vi "test Add-Find-Remove.vi"(8 "error in":errorcluster, 11 "TestCase in":refnum<class "Scripting.lvclass">) -> (0 "error out":errorcluster, 3 "TestCase out":refnum<class "Scripting.lvclass">)   [LabVIEW 2020, in "Scripting.lvclass"]
uses:
  Scripting.lvclass
  <vilib>/NI VeriStand/Custom Device API/Custom Device Item Ref.ctl
  Shared/Direction.ctl
  Shared/SDI.ctl
  Scripting.lvclass/Scripting.ctl
  Shared/Transfer Type.ctl
  <vilib>/addons/_JKI Toolkits/VI Tester/TestCase.llb/TestCase.lvclass
  Scripting/AIM/AIM ARINC 429 Scripting.lvlib
  <vilib>/NI VeriStand/Custom Device API/Custom Device API.lvlib
  C:/Program Files (x86)/National Instruments/LabVIEW 2020/vi.lib/addons/_JKI Toolkits/VI Tester/TestCase.llb/TestCase.lvclass
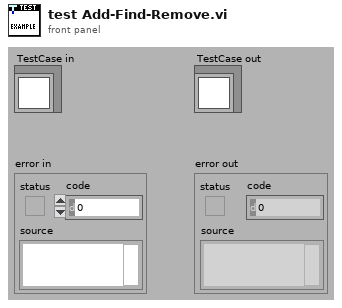
[diagram p1: front panel]
types:
  T1 = typedef "Direction.ctl" = enum16{"Rx", "Tx"}
  T2 = typedef "Custom Device API.lvlib/Custom Device Item Ref.ctl" = u64
  T3 = typedef "Transfer Type.ctl" = enum16{"Scheduled", "Acyclic", "Block", "Strobe"}
  T4 = typedef "SDI.ctl" = i32
  T5 = typedef "Custom Device API.lvlib/Custom Device Item Info.ctl" = cluster{"Name":string, "Is Channel":bool, "GUID":string, "Is Waveform":bool}
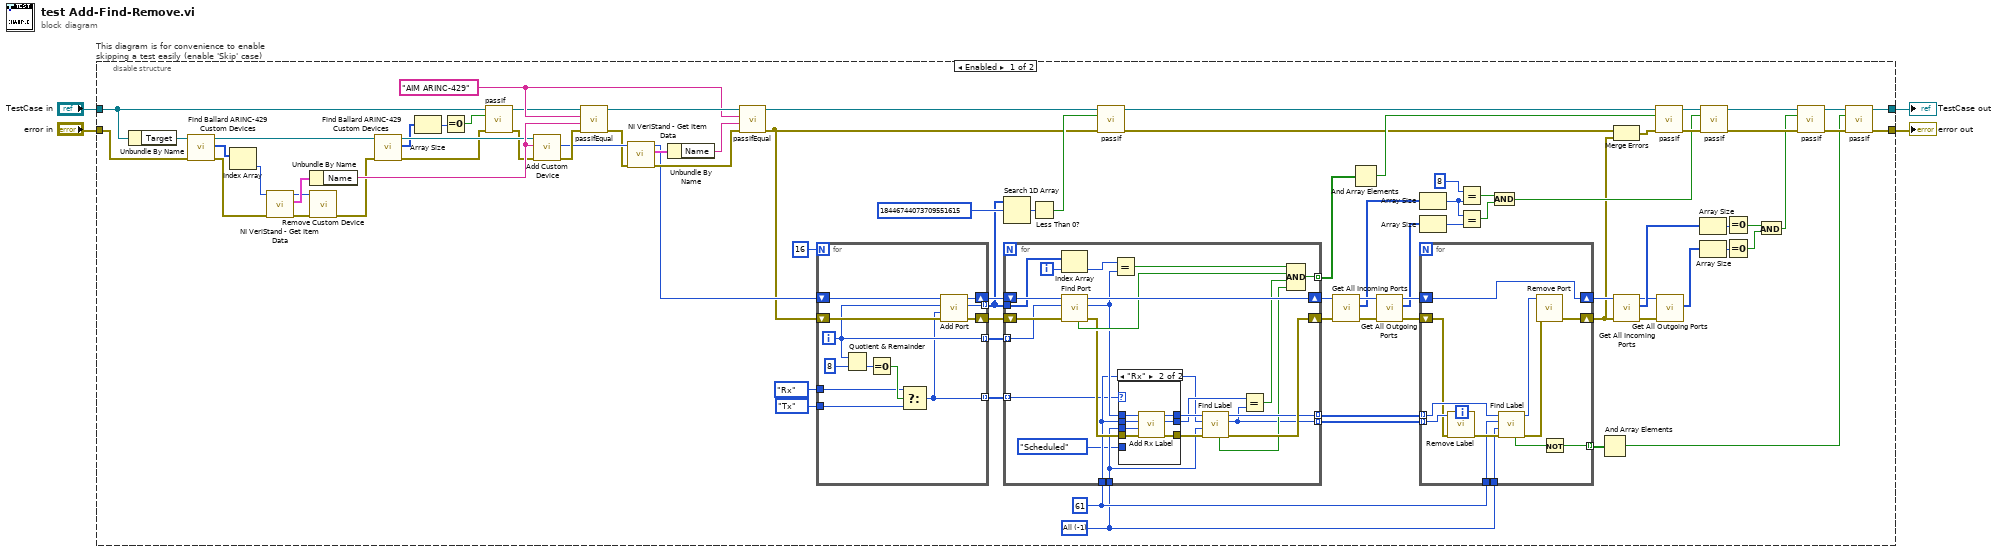
[diagram p0: block diagram]
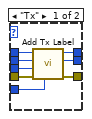
[diagram p2: hidden frame]
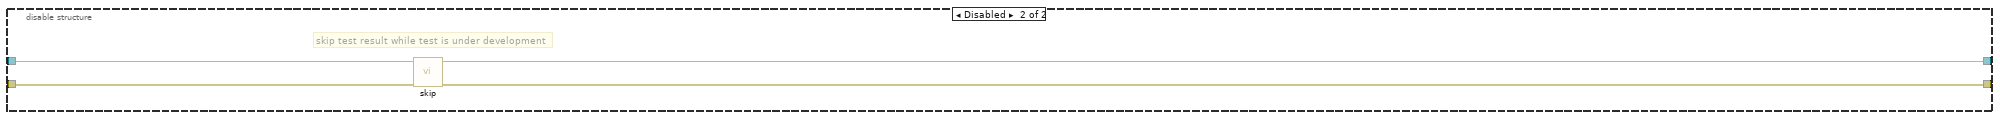
[diagram p3: hidden frame]
diagram:
  n1 = disable-structure "This diagram is for convenience to enable skipping a test easily (enable 'Skip' case)" shown="Enabled" {
    disable-tunnel: "TestCase in" -> [w69 w156]
    disable-tunnel: [w7 w154] -> w1
    disable-tunnel: [w8 w155] -> w3
    disable-tunnel: "error in" -> [w87 w153]
    frame Enabled {
      w13 = u32 61 ("label value")
      w12 = T4 -1 items=["All"=-1, "0 (b00)"=0, "1 (b01)"=1, "2 (b10)"=2, "3 (b11)"=3] ("SDI value")
      w75 = "AIM ARINC-429" ("string")
      n2 = Unbundle By Name(w69) -> ("Target"=w89:refnum<k24>)
      n3 = call "Find Ballard ARINC-429 Custom Devices.vi"("error in"=w87, "target in"=w89) -> ("error out"=w84:errorcluster, "AIM ARINC 429 custom devices"=w86:u64[], "target out"=w72:refnum<k24>)  [unwired: 7 in]
      n4 = Index Array(array=w86) -> (element=w85:u64)  [unwired: 1 in]
      n5 = call <vilib>:"NI VeriStand - Get Item Data.vi"("error in (no error)"=w84, "Item Ref in"=w85) -> ("error out"=w73:errorcluster, "Item Info"=w83:T5, "Item Ref out"=w74:T2)  [unwired: 6 in, 1 out]
      n6 = Unbundle By Name(w83) -> ("Name"=w77:string)
      n7 = call "Remove Custom Device.vi"("error in"=w73, "Ballard ARINC 429 custom device"=w74) -> ("error out"=w70:errorcluster)  [unwired: 9 in]
      n8 = call "Find Ballard ARINC-429 Custom Devices.vi"("error in"=w70, "target in"=w72) -> ("error out"=w68:errorcluster, "AIM ARINC 429 custom devices"=w65:u64[], "target out"=w71:refnum<k24>)  [unwired: 7 in]
      n9 = Array Size(array=w65) -> (size(s)=w64:i32)
      n10 = Equal To 0?(x=w64) -> (x = 0?=w63:bool)
      n11 = call-dynamic "passIf.vi"("error in (no error)"=w68, "pass"=w63, "TestCase in"=w69) -> ("error out"=w66:errorcluster, "TestCase out"=w67:refnum<class "Scripting.lvclass">)  [unwired: 7 in]
      n12 = call "Add Custom Device.vi"("error in"=w66, "name"=w77, "target in"=w71) -> ("error out"=w82:errorcluster, "Ballard ARINC 429 custom device"=w81:T2)  [unwired: 6 in, 1 out]
      n13 = call-dynamic "passIfEqual.vi"("error in (no error)"=w82, "y"=w77, "x"=w75, "TestCase in"=w67) -> ("error out"=w80:errorcluster, "TestCase out"=w88:refnum<class "Scripting.lvclass">)  [unwired: 6 in]
      n14 = call <vilib>:"NI VeriStand - Get Item Data.vi"("error in (no error)"=w80, "Item Ref in"=w81) -> ("error out"=w78:errorcluster, "Item Info"=w79:T5, "Item Ref out"=w62:T2)  [unwired: 6 in, 1 out]
      n15 = Unbundle By Name(w79) -> ("Name"=w76:string)
      n16 = call-dynamic "passIfEqual.vi"("error in (no error)"=w78, "y"=w76, "x"=w75, "TestCase in"=w88) -> ("error out"=w18:errorcluster, "TestCase out"=w21:refnum<class "Scripting.lvclass">)  [unwired: 6 in]
      n17 = for {
        N: 16 -> [_]
        shift-right: [w148] -> w61
        shift-left: w62 -> [w152]
        tunnel: [w147] -> w55 mode=indexing
        shift-right: [w145] -> w60
        shift-left: w18 -> [w146]
        tunnel: [w144] -> w59 mode=indexing
        tunnel: Direction."Rx" ("direction") -> [w143]
        tunnel: Direction."Tx" ("direction") -> [w142]
        tunnel: [w141] -> w5 mode=indexing
        i -> [w144]
        n18 = Quotient & Remainder(x=w144, y=8) -> (floor(x/y)=w150:i32)  [unwired: 1 out]
        n19 = Equal To 0?(x=w150) -> (x = 0?=w149:bool)
        n20 = Select(t=w143, s=w149, f=w142) -> (s? t:f=w141:T1)
        n21 = call "Add Port.vi"("error in"=w146, "direction"=w141, "port number"=w144, "Ballard ARINC 429 custom device in"=w152) -> ("error out"=w145:errorcluster, "port"=w147:T2, "Ballard ARINC 429 custom device out"=w148:T2)  [unwired: 5 in]
      }
      n22 = Search 1D Array(1D array=w55, element=T2 18446744073709551615 ("custom device ref out")) -> (index of element=w22:i32)  [unwired: 1 in]
      n23 = for {
        shift-right: [w124] -> w52
        shift-left: w61 -> [w125]
        tunnel: w59 -> [w122] mode=indexing
        tunnel: w55 -> [w119]
        shift-right: [w111] -> w51
        shift-left: w60 -> [w123]
        tunnel: [w110] -> w57 mode=indexing
        tunnel: [w116] -> w41 mode=indexing
        tunnel: [w106] -> w14 mode=indexing
        tunnel: w12 -> [w105]
        tunnel: w13 -> [w104]
        tunnel: w5 -> [w102] mode=indexing
        i -> [w121]
        n24 = Index Array(array=w119, index=w121) -> (element=w120:T2)
        n25 = call "Find Port.vi"("error in"=w123, "port number"=w122, "Ballard ARINC 429 custom device in"=w125) -> ("error out"=w112:errorcluster, "port"=w113:T2, "Ballard ARINC 429 custom device out"=w124:T2, "found?"=w117:bool)  [unwired: 5 in]
        n26 = Equal?(x=w120, y=w113) -> (x = y?=w118:bool)
        n27 = case shown="\"Rx\"" w102 {
          tunnel: [w133 w140] -> w115
          tunnel: [w132 w139] -> w114
          tunnel: w113 -> [w131 w138]
          tunnel: w112 -> [w130 w137]
          tunnel: [w129 w136] -> w109
          tunnel: w105 -> [w128 w135]
          tunnel: w104 -> [w127 w134]
          tunnel: Transfer_Type."Scheduled" ("transfer type") -> [w126 _]
          frame "Tx" {
            n28 = call "Add Tx Label.vi"("transfer type"=w126, "error in"=w130, "SDI value"=w128, "label value"=w127, "port in"=w131) -> ("error out"=w133:errorcluster, "label"=w129:T2, "port out"=w132:T2)  [unwired: 4 in]
          }
          frame "Rx" {
            n29 = call "Add Rx Label.vi"("error in"=w137, "SDI value"=w135, "label value"=w134, "port in"=w138) -> ("error out"=w140:errorcluster, "label"=w136:T2, "port out"=w139:T2)  [unwired: 5 in]
          }
        }
        n30 = call "Find Label.vi"("error in"=w115, "SDI value"=w105, "label value"=w104, "port in"=w114) -> ("error out"=w111:errorcluster, "label"=w106:T2, "port out"=w110:T2, "found?"=w108:bool)  [unwired: 4 in]
        n31 = Equal?(x=w109, y=w106) -> (x = y?=w107:bool)
        n32 = Compound Arithmetic op=AND(w118, w117, w107, w108) -> (w116:bool)
      }
      n33 = Less Than 0?(x=w22) -> (x < 0?=w19:bool)
      n34 = call-dynamic "passIf.vi"("error in (no error)"=w18, "pass"=w19, "TestCase in"=w21) -> ("error out"=w17:errorcluster, "TestCase out"=w20:refnum<class "Scripting.lvclass">)  [unwired: 7 in]
      n35 = call "Get All Incoming Ports.vi"("error in"=w51, "Ballard ARINC 429 custom device in"=w52) -> ("error out"=w53:errorcluster, "incoming ports"=w48:T2[], "Ballard ARINC 429 custom device out"=w54:T2)  [unwired: 7 in]
      n36 = And Array Elements(Boolean array=w41) -> (logical AND=w38:bool)
      n37 = call "Get All Outgoing Ports.vi"("error in"=w53, "Ballard ARINC 429 custom device in"=w54) -> ("error out"=w49:errorcluster, "outgoing ports"=w47:T2[], "Ballard ARINC 429 custom device out"=w50:T2)  [unwired: 7 in]
      n38 = Array Size(array=w48) -> (size(s)=w45:i32)
      n39 = Array Size(array=w47) -> (size(s)=w46:i32)
      n40 = for {
        shift-right: [w101] -> w28
        shift-left: w50 -> [w101]
        shift-right: [w100] -> w16
        shift-left: w49 -> [w97]
        tunnel: w57 -> [w98] mode=indexing
        tunnel: w14 -> [w99] mode=indexing
        tunnel: w13 -> [w95]
        tunnel: w12 -> [w94]
        tunnel: [w90] -> w11 mode=indexing
        n41 = call "Remove Label.vi"("error in"=w97, "label"=w99) -> ("error out"=w96:errorcluster)  [unwired: 9 in]
        n42 = call "Find Label.vi"("error in"=w96, "SDI value"=w94, "label value"=w95, "port in"=w98) -> ("error out"=w93:errorcluster, "port out"=w92:T2, "found?"=w91:bool)  [unwired: 4 in, 1 out]
        n43 = call "Remove Port.vi"("error in"=w93, "port"=w92) -> ("error out"=w100:errorcluster)  [unwired: 9 in]
        n44 = Not(x=w91) -> (.not. x?=w90:bool)
      }
      n45 = Equal?(x=8, y=w45) -> (x = y?=w43:bool)
      n46 = Equal?(x=w45, y=w46) -> (x = y?=w42:bool)
      n47 = And(x=w43, y=w42) -> (x .and. y?=w37:bool)
      n48 = And Array Elements(Boolean array=w11) -> (logical AND=w6:bool)
      n49 = Merge Errors(w17, w16) -> (w15:errorcluster)
      n50 = call "Get All Incoming Ports.vi"("error in"=w16, "Ballard ARINC 429 custom device in"=w28) -> ("error out"=w30:errorcluster, "incoming ports"=w31:T2[], "Ballard ARINC 429 custom device out"=w29:T2)  [unwired: 7 in]
      n51 = call-dynamic "passIf.vi"("error in (no error)"=w15, "pass"=w38, "TestCase in"=w20) -> ("error out"=w39:errorcluster, "TestCase out"=w40:refnum<class "Scripting.lvclass">)  [unwired: 7 in]
      n52 = call "Get All Outgoing Ports.vi"("error in"=w30, "Ballard ARINC 429 custom device in"=w29) -> ("outgoing ports"=w32:T2[])  [unwired: 7 in, 2 out]
      n53 = Array Size(array=w31) -> (size(s)=w34:i32)
      n54 = Array Size(array=w32) -> (size(s)=w33:i32)
      n55 = call-dynamic "passIf.vi"("error in (no error)"=w39, "pass"=w37, "TestCase in"=w40) -> ("error out"=w26:errorcluster, "TestCase out"=w27:refnum<class "Scripting.lvclass">)  [unwired: 7 in]
      n56 = Equal To 0?(x=w34) -> (x = 0?=w35:bool)
      n57 = Equal To 0?(x=w33) -> (x = 0?=w36:bool)
      n58 = And(x=w35, y=w36) -> (x .and. y?=w25:bool)
      n59 = call-dynamic "passIf.vi"("error in (no error)"=w26, "pass"=w25, "TestCase in"=w27) -> ("error out"=w10:errorcluster, "TestCase out"=w9:refnum<class "Scripting.lvclass">)  [unwired: 7 in]
      n60 = call-dynamic "passIf.vi"("error in (no error)"=w10, "pass"=w6, "TestCase in"=w9) -> ("error out"=w8:errorcluster, "TestCase out"=w7:refnum<class "Scripting.lvclass">)  [unwired: 7 in]
    }
    frame Disabled {
      # "skip test result while test is under development"
      n61 = call <vilib>:"skip.vi"("error in (no error)"=w153, "TestCase in"=w156) -> ("error out"=w155:errorcluster, "TestCase out"=w154:refnum<class "Scripting.lvclass">)  [unwired: 8 in]
    }
  }
  "error out" <- w3
  "TestCase out" <- w1
